vi "niFPGA BFGroup Twiddle Table 64 U64.vi"(7 "address":fxp<+,6,6>) -> (4 "twid real":fxp<+/-,33,2> format="%.32g", 6 "twid imag":fxp<+/-,33,2> format="%.32g")   [LabVIEW 2017]
uses:
  <vilib>/rvi/FXPMathLib/basic elements/FxpDiscreteDelay/XNode/nifxpmath_DiscreteDelay.xnode
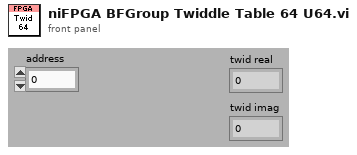
[diagram p1: front panel]
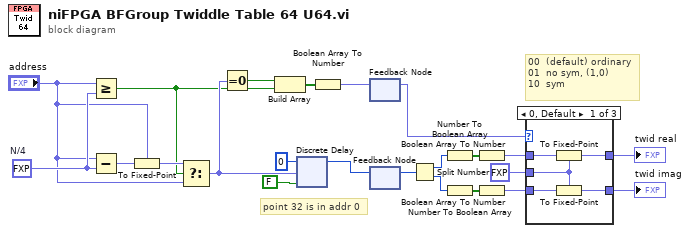
[diagram p0: block diagram]
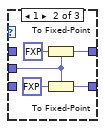
[diagram p2: hidden frame]
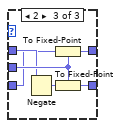
[diagram p3: hidden frame]
diagram:
  w18 = fxp<+,6,6> 32.0  # N/4
  # "point 32 is in addr 0"
  # "00  (default) ordinary\n01  no sym, (1,0)\n10  sym"
  n1 = Greater Or Equal?(x="address", y=w18) -> (x >= y?=w3:bool)
  n2 = Subtract(x="address", y=w18) -> (x-y=w17:fxp<+/-,7,7>)
  n3 = To Fixed-Point(fixed-point type="address", number=w17) -> (fixed-point=w16:fxp<+,6,6>)
  n4 = Select(t=w16, s=w3, f="address") -> (s? t:f=w6:fxp<+,6,6>)
  n5 = Equal To 0?(x=w6) -> (x = 0?=w2:bool)
  n6 = Build Array(w2, w3) -> (w4:bool[])
  n7 = xnode "Discrete Delay"("D"=u64 0, "n-1[0..31]"=w6, "enable"=FALSE) -> ("Q"=w5:u64)
  n8 = Boolean Array To Number(Boolean array=w4) -> (number=w1:fxp<+,2,2>)
  n9 = feedback-in #1(w1) -> ()
  n10 = feedback #1() -> (w9:fxp<+,2,2>)  [unwired: 1 out]
  n11 = feedback-in #2(w5) -> ()
  n12 = feedback #2() -> (w19:u64)  [unwired: 1 out]
  n13 = Split Number(x=w19) -> (hi(x)=w22:u32, lo(x)=w20:u32)
  n14 = Number To Boolean Array(number=w22) -> (Boolean array=w23:bool[])
  n15 = Number To Boolean Array(number=w20) -> (Boolean array=w21:bool[])
  n16 = Boolean Array To Number(Boolean array=w23) -> (number=w13:fxp<+/-,32,1>)
  n17 = Boolean Array To Number(Boolean array=w21) -> (number=w11:fxp<+/-,32,1>)
  n18 = case shown="0, Default" w9 {
    tunnel: w13 -> [w28 _ w36]
    tunnel: [w27 w32 w34] -> w12
    tunnel: w11 -> [w26 _ w35]
    tunnel: [w25 w30 w39] -> w10
    tunnel: fxp<+/-,33,2> 0.0 ("fixed-point type") -> [w24 w29 w37]
    frame 0, Default {
      n19 = To Fixed-Point(fixed-point type=w24, number=w28) -> (fixed-point=w27:fxp<+/-,33,2>)
      n20 = To Fixed-Point(fixed-point type=w24, number=w26) -> (fixed-point=w25:fxp<+/-,33,2>)
    }
    frame 1 {
      n21 = To Fixed-Point(fixed-point type=w29, number=fxp<+,1,1> 1.0 ("fixed-point type")) -> (fixed-point=w32:fxp<+/-,33,2>)
      n22 = To Fixed-Point(fixed-point type=w29, number=fxp<+,1,1> 0.0 ("fixed-point type")) -> (fixed-point=w30:fxp<+/-,33,2>)
    }
    frame 2 {
      n23 = Negate(x=w36) -> (-x=w38:fxp<+/-,33,2>)
      n24 = To Fixed-Point(fixed-point type=w37, number=w35) -> (fixed-point=w34:fxp<+/-,33,2>)
      n25 = To Fixed-Point(fixed-point type=w37, number=w38) -> (fixed-point=w39:fxp<+/-,33,2>)
    }
  }
  "twid real" <- w12
  "twid imag" <- w10
